vi "example test.vi"() -> ()   [LabVIEW 2013, in "tdms logger tests.lvlib"]
uses:
  tdms logger tests.lvlib
  <vilib>/NI/Tag Bus/tag/Data Type.ctl
  <vilib>/NI/Tag Bus Module Framework/channel/channel classification.ctl
  configuration/TDMS datalogger configuration.lvclass
  execution/TDMS datalogger runtime.lvclass
  configuration/TDMS datalogger configuration.lvclass/TDMS datalogger configuration.ctl
  <vilib>/NI/Tag Bus/dictionary/data dictionary.lvclass/data dictionary.ctl
  <vilib>/NI/Tag Bus/dictionary/lookup polymorphs/locate double.vi
  <vilib>/NI/Tag Bus/table/data polymorphs/write one/write Double.vi
  configuration/Write channels.vi
  configuration/Write backup directory.vi
  configuration/Write Path.vi
  <vilib>/NI/Tag Bus/dictionary/search/find data index.vi
  <vilib>/NI/Tag Bus/dictionary/search/search string list.vi
  <vilib>/NI/Tag Bus/dictionary/tag not found.vi
  <vilib>/NI/Tag Bus Module Framework/channel/TBM channel.lvclass
  <vilib>/NI/Tag Bus/tag/tag descriptor.lvclass
  <vilib>/NI/Tag Bus/dictionary/data dictionary.lvclass
  <vilib>/NI/Tag Bus/table/data table.lvlib
  <vilib>/NI/Configuration Framework/serializable configuration/NISE_CEF_serializable configuration.lvclass
panel:
  out "final error":errorcluster
  out "output error":errorcluster
  out "output lookup error":errorcluster
  out "init error":errorcluster
  out "correct execution settings":bool
  out "serialization problem":errorcluster
  out "invalid configuration":errorcluster
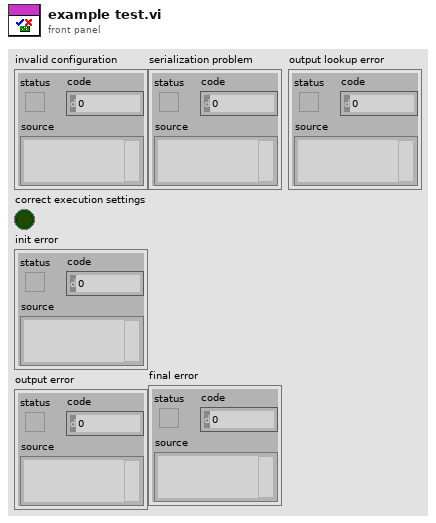
[diagram p1: front panel]
types:
  T1 = typedef "TBM channel.lvclass/channel classification.ctl" = enum16{"input data", "output data", "processing parameter", "processing result"}
  T2 = typedef "tag bus.lvlib/tag descriptor.lvclass/Data Type.ctl" = enum16{"Double", "Single", "I64", "I32", "I16", "I8", "U64", "U32", "U16", "U8", "Boolean", "String", "Array of Double", "Array of Single", "Array of I64", "Array of I32", "Array of I16", "Array of I8", "Array of U64", "Array of U32", "Array of U16", "Array of U8", "Array of Boolean", "Array of String"}
  T3 = typedef "TBM channel.lvclass/data tables.ctl" = cluster{"input data":T4, "processing parameter":T4, "processing result":T4, "output data":T4}
  T4 = typedef "tag bus.lvlib/dictionary table pair.ctl" = cluster{"data dictionary":refnum<class "data dictionary.lvclass">, "data table":T5}
  T5 = typedef "tag bus.lvlib/data table.lvlib/data table.ctl" = cluster{"Double":dbl[], "Single":sgl[], "I64":i64[], "I32":i32[], "I16":i16[], "I8":i8[], "U64":u64[], "U32":u32[], "U16":u16[], "U8":u8[], "Boolean":bool[], "String":string[], "Array of Double":cluster{"DBL Array":dbl[]}[], "Array of Single":cluster{"SGL Array":sgl[]}[], "Array of I64":cluster{"I64 Array":i64[]}[], "Array of I32":cluster{"I32 Array":i32[]}[], "Array of I16":cluster{"I16 Array":i16[]}[], "Array of I8":cluster{"I8 Array":i8[]}[], "Array of U64":cluster{"U64 Array":u64[]}[], "Array of U32":cluster{"U32 Array":u32[]}[], "Array of U16":cluster{"U16 Array":u16[]}[], "Array of U8":cluster{"U8 Array":u8[]}[], "Array of Boolean":cluster{"Boolean Array":bool[]}[], "Array of String":cluster{"String Array":string[]}[]}
  T6 = typedef "TBM module execution interface.lvclass/execution settings.ctl" = cluster{"reads inputs":bool, "processes data":bool, "writes outputs":bool}
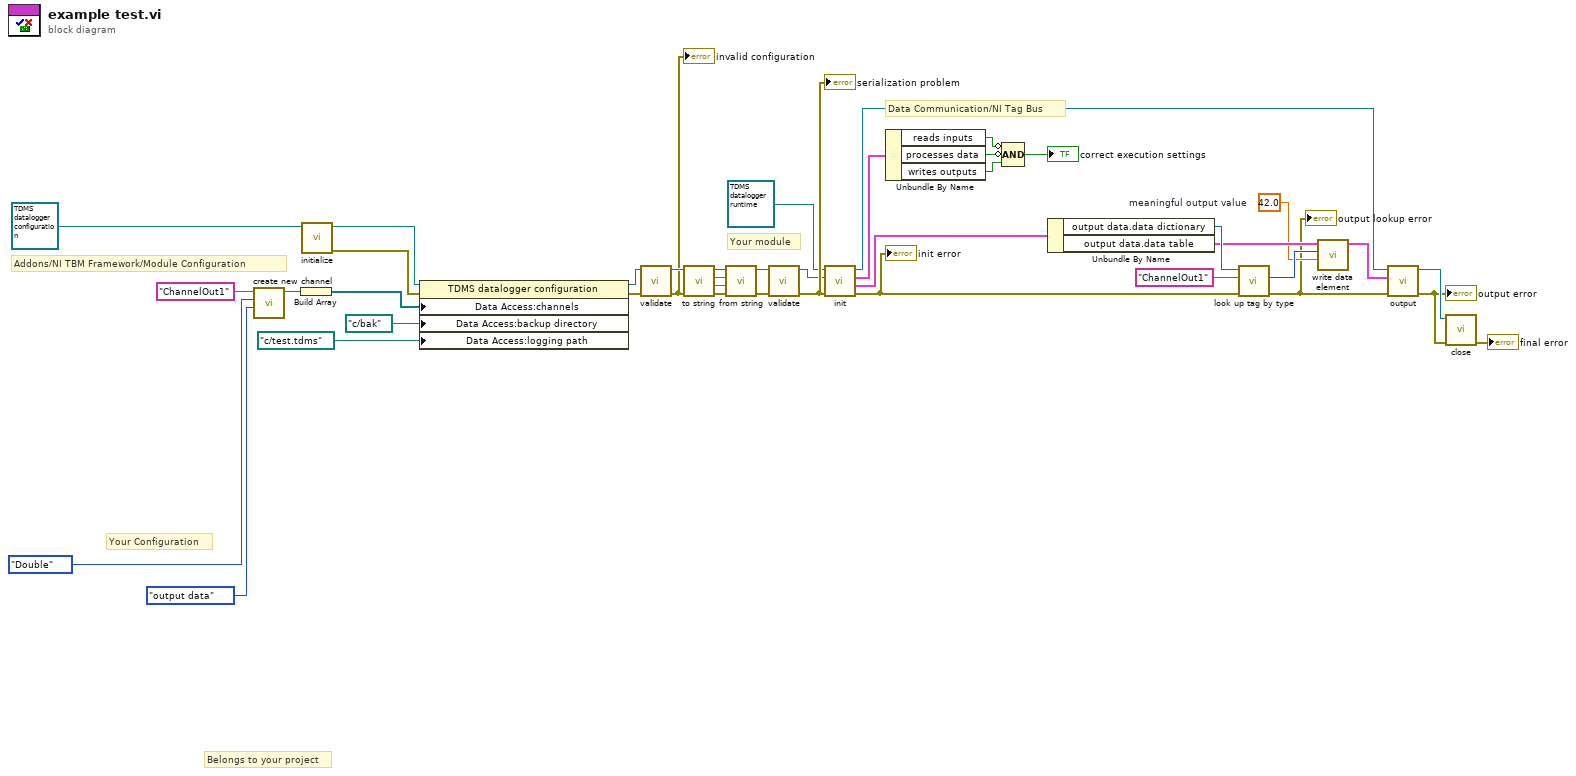
[diagram p0: block diagram]
diagram:
  w16 = 42.0  # meaningful output value
  # "Data Communication/NI Tag Bus"
  # "Your module"
  # "Your Configuration"
  # "Addons/NI TBM Framework/Module Configuration"
  # "Belongs to your project"
  n1 = call <vilib>:"create new channel.vi"("channel classification"=channel_classification."output data", "data type"=Data_Type."Double", "channel name"="ChannelOut1") -> ("channel"=w10:refnum<class "TBM channel.lvclass">)  [unwired: 8 in]
  n2 = Build Array(w10) -> (w7:refnum<class "TBM channel.lvclass">[])
  n3 = call <vilib>:"initialize.vi"("configuration in"=refnum<class "TDMS datalogger configuration.lvclass"> refnum ("TDMS datalogger configuration")) -> ("error out"=w1:errorcluster, "configuration out"=w2:refnum<class "TDMS datalogger configuration.lvclass">)  [unwired: 8 in, 1 out]
  n4 = property class="TDMS datalogger configuration"(reference=w2, error in=w1, "Data Access:channels"=w7, "Data Access:backup directory"=path "c:/bak" ("backup directory"), "Data Access:logging path"=path "c:/test.tdms" ("logging path")) -> (reference out=w9:refnum<class "TDMS datalogger configuration.lvclass">, error out=w8:errorcluster)
  n5 = call-dynamic "validate.vi"("error in"=w8, "TDMS datalogger configuration in"=w9) -> ("error out"=w37:errorcluster, "TDMS datalogger configuration out"=w38:refnum<class "TDMS datalogger configuration.lvclass">)  [unwired: 8 in]
  "invalid configuration" <- w37
  n6 = call-dynamic "to string.vi"("error in"=w37, "TDMS datalogger configuration in"=w38) -> ("error out"=w33:errorcluster, "data"=w34:string, "version"=w35:string, "TDMS datalogger configuration out"=w36:refnum<class "TDMS datalogger configuration.lvclass">)  [unwired: 6 in]
  n7 = call-dynamic "from string.vi"("error in"=w33, "data"=w34, "version"=w35, "TDMS datalogger configuration in"=w36) -> ("error out"=w31:errorcluster, "TDMS datalogger configuration out"=w32:refnum<class "TDMS datalogger configuration.lvclass">)  [unwired: 6 in]
  n8 = call-dynamic "validate.vi"("error in"=w31, "TDMS datalogger configuration in"=w32) -> ("error out"=w30:errorcluster, "TDMS datalogger configuration out"=w29:refnum<class "TDMS datalogger configuration.lvclass">)  [unwired: 8 in]
  "serialization problem" <- w30
  n9 = call-dynamic "init.vi"("error in"=w30, "TBM module configuration in"=w29, "TDMS datalogger runtime in"=refnum<class "TDMS datalogger runtime.lvclass"> refnum ("TDMS datalogger runtime")) -> ("error out"=w22:errorcluster, "data allocations"=w23:T3, "execution settings"=w28:T6, "TDMS datalogger runtime out"=w21:refnum<class "TDMS datalogger runtime.lvclass">)  [unwired: 5 in]
  "init error" <- w22
  n10 = Unbundle By Name(w28) -> ("reads inputs"=w25:bool, "processes data"=w27:bool, "writes outputs"=w26:bool)
  n11 = Compound Arithmetic op=AND(invert w25, invert w27, w26) -> (→"correct execution settings":bool)
  n12 = Unbundle By Name(w23) -> ("output data.data dictionary"=w20:refnum<class "data dictionary.lvclass">, "output data.data table"=w17:T5)
  n13 = call-poly <vilib>:"look up tag by type.vi"("error in"=w22, "name"="ChannelOut1" ("channel name"), "data dictionary in"=w20) -> ("error out"=w15:errorcluster, "index"=w18:i32)  [unwired: 6 in, 1 out]
  "output lookup error" <- w15
  n14 = call-poly <vilib>:"write data element.vi"("value"=w16, "index"=w18, "data table in"=w17) -> ("data table out"=w14:T5)  [unwired: 8 in]
  n15 = call-dynamic "output.vi"("error in"=w15, "data table in"=w14, "TDMS datalogger runtime in"=w21) -> ("error out"=w12:errorcluster, "TDMS datalogger runtime out"=w13:refnum<class "TDMS datalogger runtime.lvclass">)  [unwired: 6 in, 1 out]
  "output error" <- w12
  n16 = call-dynamic "close.vi"("error in"=w12, "TDMS datalogger runtime in"=w13) -> ("error out"=→"final error":errorcluster)  [unwired: 9 in]
